vi "Falling Edge.vi"(11 "signal in":bool) -> (3 "falling edge?":bool)   [LabVIEW 2013, in "I2S-TDM.lvlib"]
uses:
  I2S-TDM.lvlib
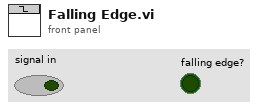
[diagram p1: front panel]
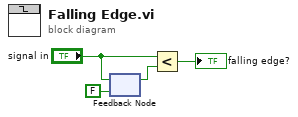
[diagram p0: block diagram]
diagram:
  n1 = feedback-in #1("signal in") -> ()
  n2 = feedback #1(FALSE ("signal in")) -> (w3:bool)
  n3 = Less?(x="signal in", y=w3) -> (x < y?=→"falling edge?":bool)
